vi "Get_TrackFrames.vi"(8 "error in":errorcluster, 11 "camera handle in":u64) -> (0 "error out":errorcluster, 1 "TrackFrames":bool, 3 "camera handle out":u64)   [LabVIEW 2019, in "PICam.lvlib"]
doc: "Requests the time the sensor is exposed in milliseconds (mS)."
uses:
  PICam.lvlib
  Picam64.dll   
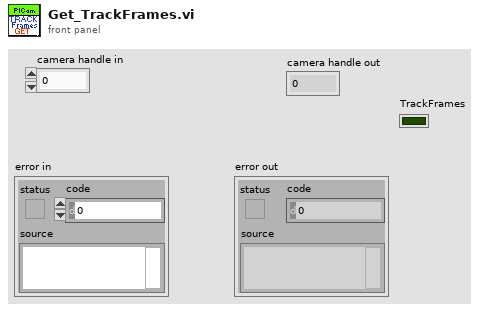
[diagram p1: front panel]
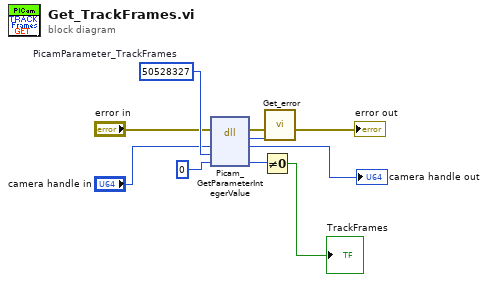
[diagram p0: block diagram]
diagram:
  w6 = u32 50528327  # PicamParameter_TrackFrames
  n1 = dll-call lib="Picam32.dll" fn="Picam_GetParameterIntegerValue"(error in="error in", "camera"="camera handle in", "PicamParameter"=w6, "TrackFrames"=0) -> (error out=w10:errorcluster, "return type"=w9:i32, "camera"=→"camera handle out":u64, "TrackFrames"=w2:i32)  [unwired: 3 in, 1 out]
  n2 = Not Equal To 0?(x=w2) -> (x != 0?=→"TrackFrames":bool)
  n3 = call "Get_error.vi"("PICam_Error"=w9, "error in (no error)"=w10) -> ("error out"=→"error out":errorcluster)  [unwired: 9 in]
